vi "Konwersja_kanalow_z_pliku.vi"(9 "Kanal 2":i32, 10 "Kanal 1":i32, 11 "Typ rejestracji":T1) -> (2 "Kanaly":i32[](array[numeric]))   [LabVIEW 2014]
uses:
  Kontrolki/GUI/RejWol_typ.ctl
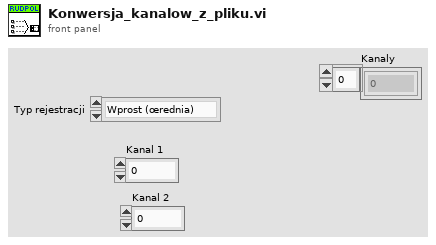
[diagram p1: front panel]
types:
  T1 = typedef "RejWol_typ.ctl" = enum16{"Wprost (œrednia)", "Modu³ (œr. wypr)", "Kwadrat (skuteczna)", "Iloczyn", "Faza"}
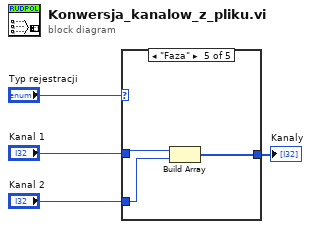
[diagram p0: block diagram]
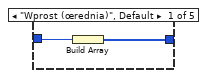
[diagram p2: hidden frame]
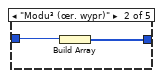
[diagram p3: hidden frame]
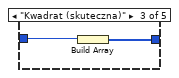
[diagram p4: hidden frame]
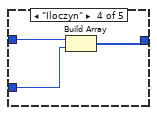
[diagram p5: hidden frame]
diagram:
  n1 = case shown="\"Faza\"" "Typ rejestracji" {
    tunnel: "Kanal 1" -> [w6 w8 w10 w13 w16]
    tunnel: "Kanal 2" -> [_ _ _ w12 w15]
    tunnel: [w5 w7 w9 w11 w14] -> w1
    frame "Wprost (œrednia)", Default {
      n2 = Build Array(w6) -> (w5:i32[])
    }
    frame "Modu³ (œr. wypr)" {
      n3 = Build Array(w8) -> (w7:i32[])
    }
    frame "Kwadrat (skuteczna)" {
      n4 = Build Array(w10) -> (w9:i32[])
    }
    frame "Iloczyn" {
      n5 = Build Array(w13, w12) -> (w11:i32[])
    }
    frame "Faza" {
      n6 = Build Array(w16, w15) -> (w14:i32[])
    }
  }
  "Kanaly" <- w1
